vi "DHE_TP.vi"(0 "refnum":i32, 5 "Command":string, 7 "physical unit":string, 9 "swhitches":string[](array[string]), 11 "error in (no error)":errorcluster, 12 "switch arguments":string[](array[string]), 13 "Database RefNum in":T1) -> (4 "refnum out":i32, 6 "response":string, 15 "error out":errorcluster)   [LabVIEW 2016]
uses:
  DBSHAND/private/vis/DatabaseHand_RefNum.ctl
  DHE_TP_action.ctl
panel:
  in  "suscribed?":bool
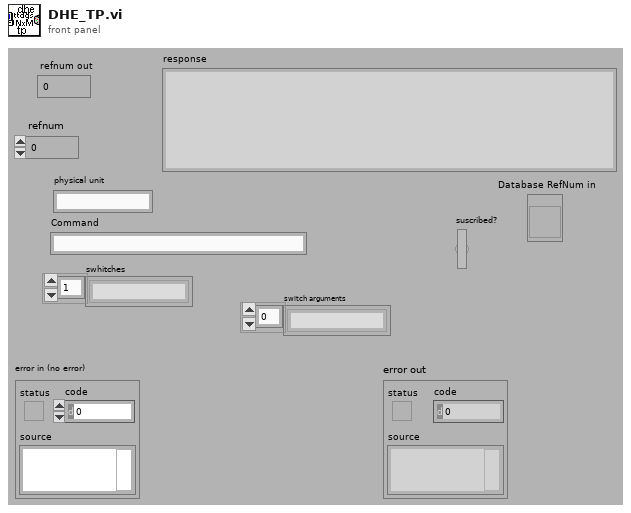
[diagram p1: front panel]
types:
  T1 = typedef "DatabaseHand_RefNum.ctl" = refnum<vi>
  T2 = typedef "DHE_TP_action.ctl" = enum16{"READ FROM FILE", "GET ALL", "FIND BY NAME", "FIND BY TYPE", "SET VALUE", "CLEAN", "CHANGE", "GET EXPUPDATE"}
  T3 = enum16{"convert", "read from file", "get", "clear all", "get all"}
  T4 = enum16{"convert", "read from file", "get", "clear all", "get all", "delete"}
  T5 = typedef "CMN_ContStatus.ctl" = cluster{"Response":string, "power":bool, "shutter":bool, "artifdata":bool, "idlemode":bool, "reset":bool, "gain":u8, "speed":u8, "resetPCI":bool, "autoshutter":bool, "TempSetPoint":i32, "multipleextensions":bool, "displayImage":bool, "coadding":bool, "images being coadded":i32, "Operation Mode":enum16{"normal", "coadd", "fawler"}, "frames to write":cluster{"subs":bool, "reset":bool, "exposed":bool}, "fawler samples":i32, "write auto":bool, "datatype":string, "frames to display":cluster{"subs":bool, "reset":bool, "exposed":bool}, "sur":i32, "autoclear":bool}
  T6 = enum16{"Idle", "Exposing", "Paused", "AbortExp", "Reading", "AbortRead", "FinishedReading", "Resetting", "Reducing", "Initializing"}
  T7 = typedef "DHE_TP.ctl" = cluster{"name":string, "type":string, "R_algor":string[], "board":string, "memory":string, "address":i32, "value":string, "Limits":T8, "unit":string, "params":string, "permissions":string, "W_algor":string[], "description":string, "err_count":i32, "max_err":i32, "read":bool, "lowrej":dbl, "hirej":dbl, "expupd":bool}
  T8 = typedef "DHE_TPLimits.ctl" = cluster{"upper":dbl, "Lower":dbl, "InRange":bool, "nominal":dbl}
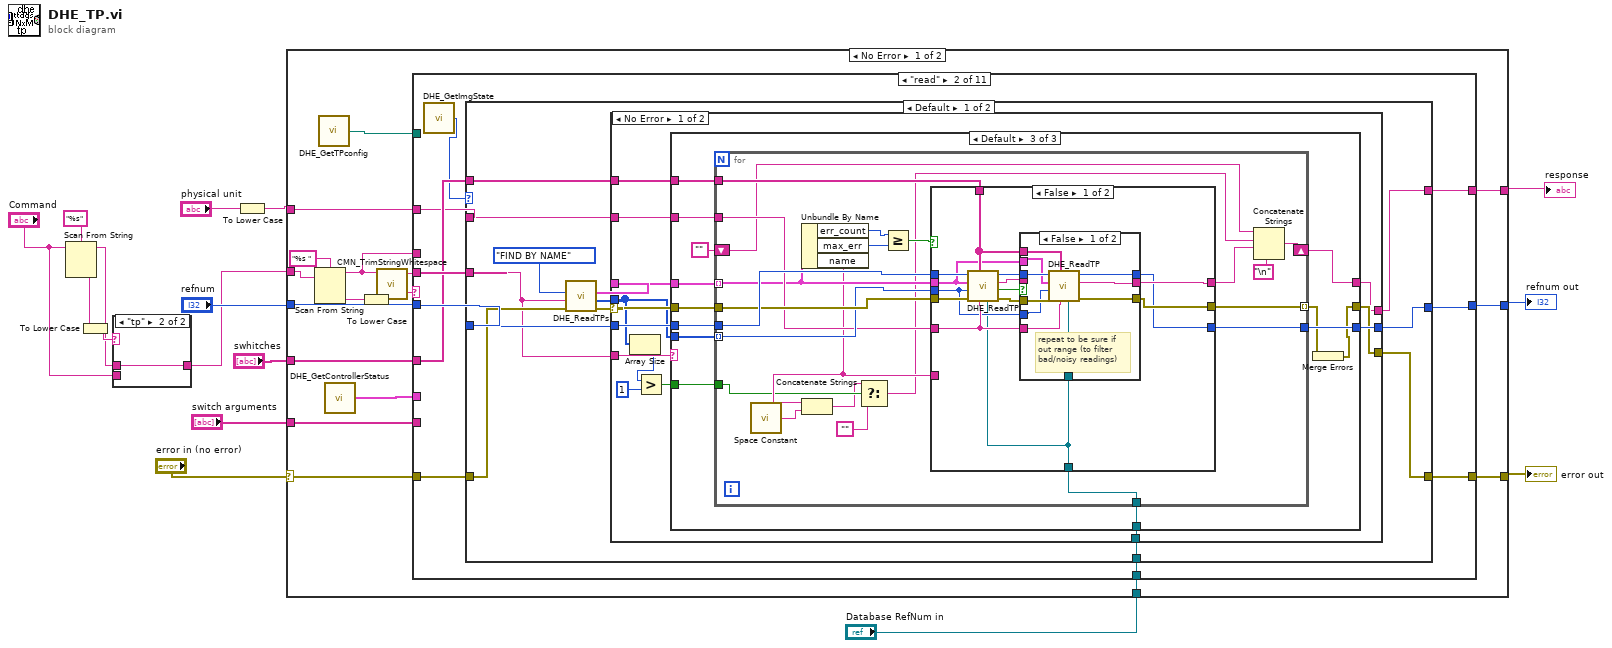
[diagram p0: block diagram]
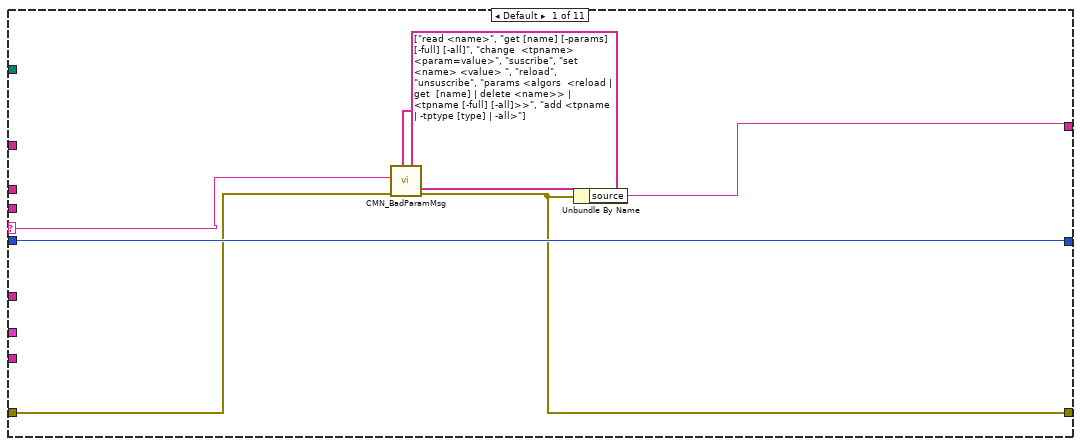
[diagram p3: hidden frame]
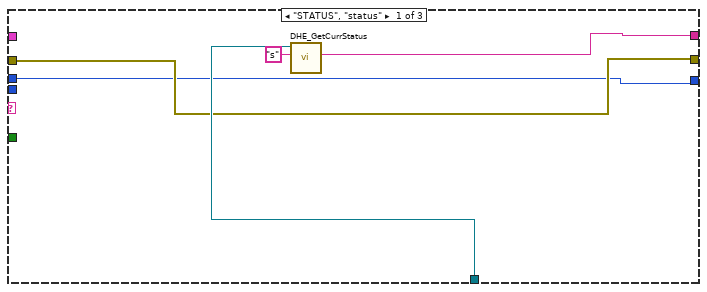
[diagram p4: hidden frame]
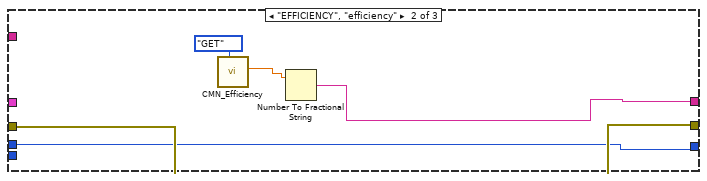
[diagram p5: hidden frame]
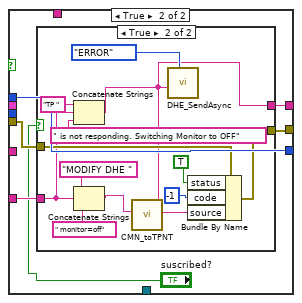
[diagram p7: hidden frame]
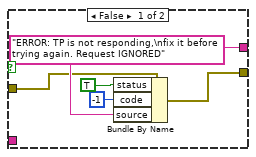
[diagram p8: hidden frame]
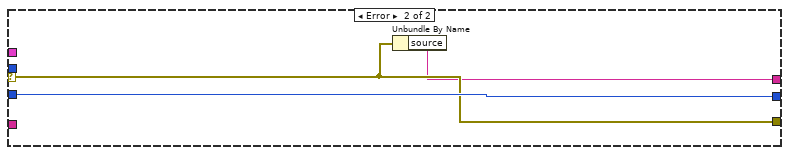
[diagram p9: hidden frame]
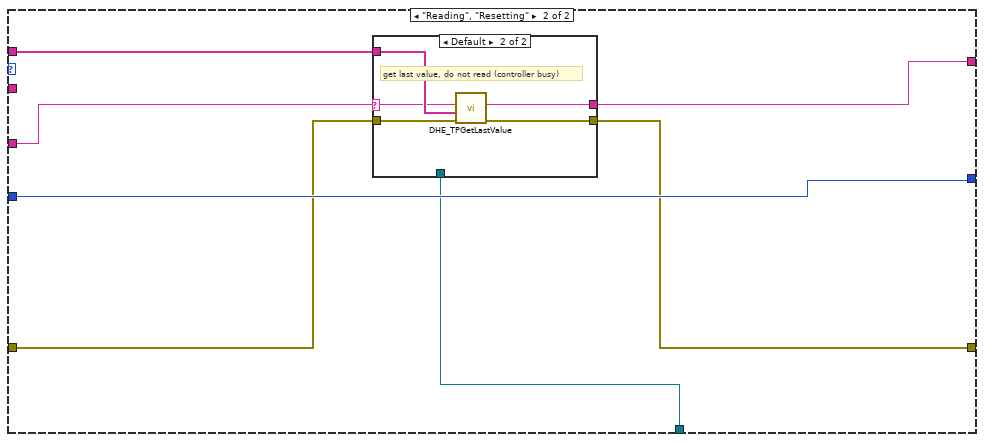
[diagram p10: hidden frame]
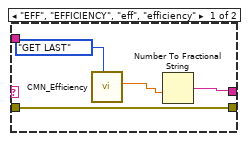
[diagram p11: hidden frame]
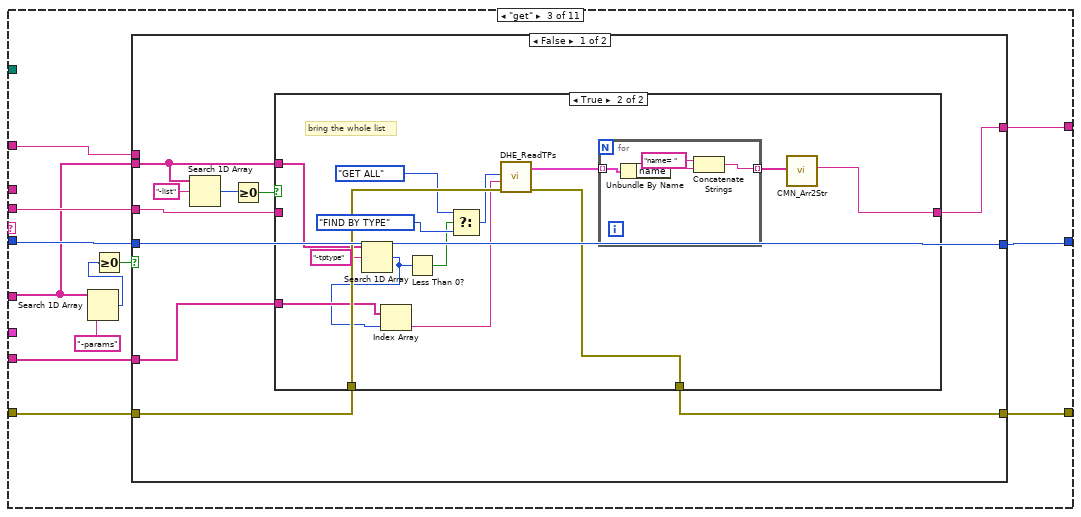
[diagram p12: hidden frame]
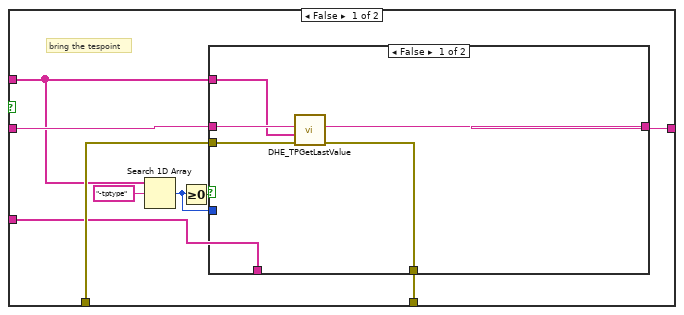
[diagram p13: hidden frame]
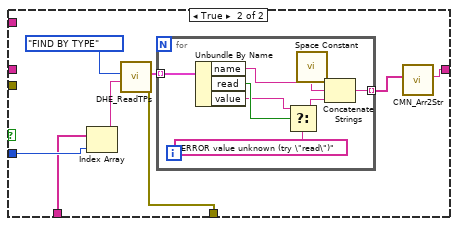
[diagram p14: hidden frame]
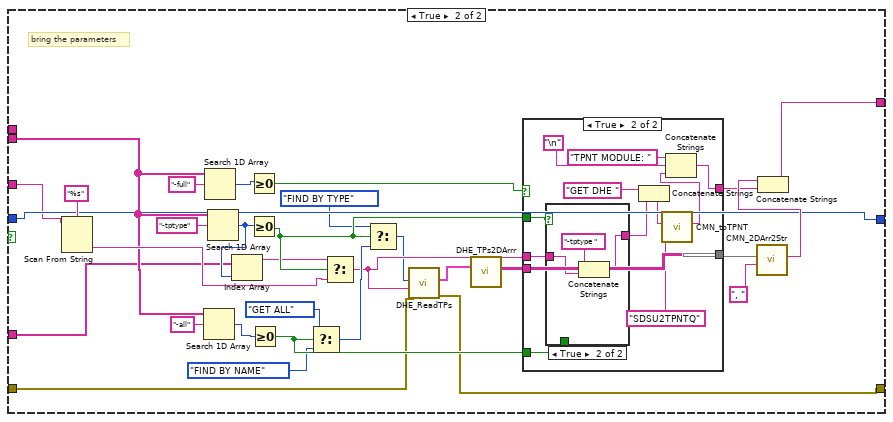
[diagram p15: hidden frame]
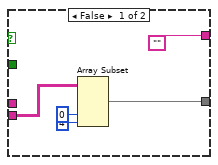
[diagram p16: hidden frame]
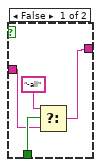
[diagram p17: hidden frame]
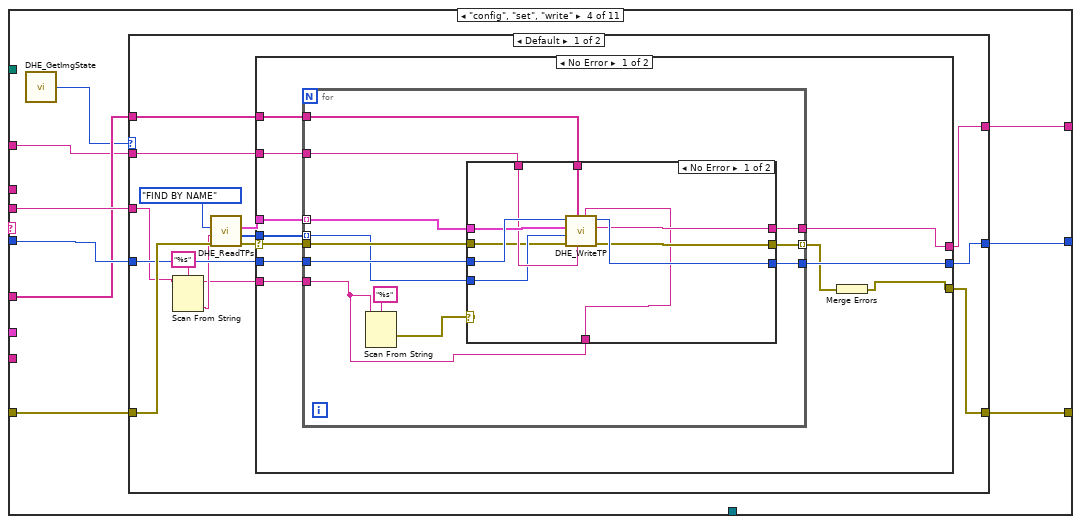
[diagram p18: hidden frame]
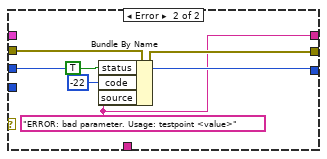
[diagram p19: hidden frame]
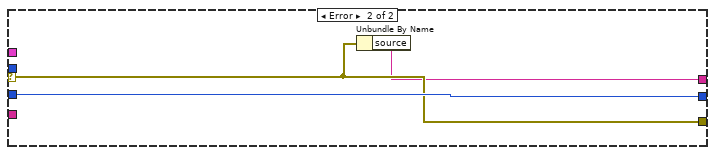
[diagram p20: hidden frame]
diagram:
  n1 = Scan From String(format string="%s", input string="Command") -> (remaining string=w3:string, output 1=w5:string)  [unwired: 2 in, 3 out]
  n2 = To Lower Case(string=w5) -> (all lower case string=w4:string)
  n3 = case shown="\"tp\"" w4 {
    tunnel: w3 -> [_ w18]
    tunnel: [w17 w18] -> w2
    tunnel: "Command" -> [w17 _]
    frame Default {
    }
    frame "tp" {
    }
  }
  n4 = To Lower Case(string="physical unit") -> (all lower case string=w12:string)
  n5 = case shown="No Error" "error in (no error)" {
    selector: "error in (no error)" -> [w22 w635]
    tunnel: [w35 w635] -> w14
    tunnel: "refnum" -> [w34 w637]
    tunnel: [w33 w637] -> w16
    tunnel: w2 -> [w26 _]
    tunnel: w12 -> [w25 _]
    tunnel: [w24 w636] -> w11
    tunnel: "swhitches" -> [w23 _]
    tunnel: "switch arguments" -> [w21 _]
    tunnel: "Database RefNum in" -> [w20 _]
    frame No Error {
      n6 = Scan From String(format string="%s " ("Format String"), input string=w26) -> (remaining string=w28:string, output 1=w29:string)  [unwired: 2 in, 3 out]
      n7 = call "DHE_GetTPconfig.vi"() -> ("DHE_TPcfg"=w19:path)  [unwired: 9 out]
      n8 = call "DHE_GetControllerStatus.vi"() -> ("ControllerStatus"=w27:T5)  [unwired: 11 out]
      n9 = To Lower Case(string=w29) -> (all lower case string=w30:string)
      n10 = call "CMN_TrimStringWhitespace.vi"("string"=w28) -> ("trimmed string"=w31:string)  [unwired: 1 in, 8 out]
      n11 = case shown="\"read\"" w30 {
        selector: w30 -> [w39 _ _ _ _ _ _ _ _ _ _]
        tunnel: w22 -> [w40 w50 w194 w325 _ w461 w472 w481 w505 w609 w634]
        tunnel: [w38 w48 w193 w323 w395 w454 w466 w478 w504 w594 w634] -> w35
        tunnel: w34 -> [w41 w46 w197 w321 w396 w460 w471 w493 w503 w608 w633]
        tunnel: [w41 w49 w204 w324 w396 w460 w471 w493 w503 w608 w633] -> w33
        tunnel: w31 -> [_ w51 w198 w326 w408 w462 _ _ w500 w593 _]
        tunnel: w27 -> [_ _ _ _ _ _ _ _ _ _ _]
        tunnel: w28 -> [_ _ _ _ _ _ _ _ _ _ _]
        tunnel: w25 -> [_ w44 w199 w319 _ _ _ _ _ _ _]
        tunnel: [w37 w47 w203 w322 w391 w459 w464 w492 w501 w607 "module= DHE, prefix= DHE TP, updatecapable= yes, hardware=  DHE hardware controller"] -> w24
        tunnel: w23 -> [_ w45 w196 w320 w399 _ _ _ w502 w598 _]
        tunnel: w21 -> [_ _ w195 _ w398 _ _ _ w506 w610 _]
        tunnel: w19 -> [_ _ _ _ _ _ w473 w479 _ _ _]
        tunnel: w20 -> [_ w43 _ _ _ _ _ _ _ _ _]
        frame Default {
          n12 = call "CMN_BadParamMsg.vi"("valid params"=string[] ["read <name>", "get [name] [-params] [-full] [-all]", "change  <tpname> <param=value>", "suscribe", "set <name> <value> ", "reload", "unsuscribe", "params <algors  <reload | get  [name] | delete <name>> | <tpname [-full] [-all]>>", "add <tpname | -tptype [type] | -all>"], "error in (no error)"=w40, "parameter"=w39) -> ("error out"=w38:errorcluster)  [unwired: 1 in, 7 out]
          n13 = Unbundle By Name(w38) -> ("source"=w37:string)
        }
        frame "read" {
          n14 = call "DHE_GetImgState.vi"() -> ("DHE_ImgState"=w42:T6)  [unwired: 9 out]
          n15 = case shown="Default" w42 {
            tunnel: w51 -> [w53 w178]
            tunnel: w50 -> [w64 w181]
            tunnel: [w63 w183] -> w49
            tunnel: [w62 w180] -> w48
            tunnel: [w61 w179] -> w47
            tunnel: w46 -> [w60 w183]
            tunnel: w45 -> [w59 w182]
            tunnel: w44 -> [w58 _]
            tunnel: w43 -> [w57 w177]
            frame Default {
              n16 = call "DHE_ReadTPs.vi"("error in (no error)"=w64, "argument"=w53, "action"=DHE_TP_action."FIND BY NAME") -> ("error out"=w56:errorcluster, "index"=w54:i32[], "TPs"=w55:T7[])  [unwired: 4 in, 2 out]
              n17 = case shown="No Error" w56 {
                selector: w56 -> [w76 w175]
                tunnel: w55 -> [w74 _]
                tunnel: w60 -> [w78 w176]
                tunnel: [w77 w176] -> w63
                tunnel: [w75 w175] -> w62
                tunnel: [w73 w174] -> w61
                tunnel: w59 -> [w72 _]
                tunnel: w58 -> [w71 _]
                tunnel: w54 -> [w68 _]
                tunnel: w57 -> [w70 _]
                tunnel: w53 -> [w69 _]
                frame No Error {
                  n18 = Array Size(array=w68) -> (size(s)=w67:i32)
                  n19 = Greater?(x=w67, y=1) -> (0:w65:bool)
                  n20 = case shown="Default" w69 {
                    tunnel: w78 -> [w79 w87 w101]
                    tunnel: [w79 w87 w100] -> w77
                    tunnel: w76 -> [w80 w88 w99]
                    tunnel: [w80 w88 w92] -> w75
                    tunnel: w74 -> [_ _ w98]
                    tunnel: w68 -> [_ _ w97]
                    tunnel: [w81 w84 w91] -> w73
                    tunnel: w72 -> [_ _ w96]
                    tunnel: w71 -> [_ _ w95]
                    tunnel: w70 -> [w83 _ w94]
                    tunnel: w65 -> [_ _ w89]
                    frame "STATUS", "status" {
                      n21 = call "DHE_GetCurrStatus.vi"("phys. unit"="s", "Databse Ref"=w83) -> ("progress"=w81:string)  [unwired: 9 out]
                    }
                    frame "EFFICIENCY", "efficiency" {
                      n22 = call "CMN_Efficiency.vi"("Action"=enum16{"ADD", "CLEAR", "GET"}."GET") -> ("efficency"=w85:dbl)  [unwired: 3 in, 7 out]
                      n23 = Number To Fractional String(number=w85) -> (F-format string=w84:string)  [unwired: 3 out]
                    }
                    frame Default {
                      n24 = for {
                        tunnel: w101 -> [w123]
                        tunnel: [w109] -> w100
                        tunnel: w99 -> [w122]
                        tunnel: [w121] -> w93 mode=indexing
                        tunnel: w98 -> [w113] mode=indexing
                        tunnel: w97 -> [w120] mode=indexing
                        tunnel: w96 -> [w119]
                        tunnel: w95 -> [w118]
                        tunnel: w94 -> [w114]
                        shift-right: [w110] -> w91
                        shift-left: "" -> [w108]
                        tunnel: w89 -> [w105]
                        n25 = call <vilib>:"Space Constant.vi"() -> ("String"=w106:string)
                        n26 = Unbundle By Name(w113) -> ("err_count"=w117:i32, "max_err"=w116:i32, "name"=w107:string)
                        n27 = Concatenate Strings(w107, w106) -> (w104:string)
                        n28 = Select(t=w104, s=w105, f="") -> (s? t:f=w102:string)
                        n29 = Greater Or Equal?(x=w117, y=w116) -> (x >= y?=w115:bool)
                        n30 = case shown="False" w115 {
                          tunnel: w123 -> [w137 w156]
                          tunnel: [w129 w156] -> w109
                          tunnel: w122 -> [w136 w154]
                          tunnel: [w133 w153] -> w121
                          tunnel: w120 -> [w125 _]
                          tunnel: [w131 w155] -> w112
                          tunnel: w119 -> [w128 _]
                          tunnel: w118 -> [w127 _]
                          tunnel: w113 -> [w126 _]
                          tunnel: w107 -> [_ w152]
                          tunnel: w114 -> [w124 _]
                          frame False {
                            n31 = call "DHE_ReadTP.vi"("Database RefNum in"=w124, "phys. unit"=w127, "switches"=w128, "error in (no error)"=w136, "index in"=w125, "TP In"=w126, "refnum"=w137) -> ("error out"=w134:errorcluster, "In Range?"=w135:bool, "response"=w132:string, "refnum out"=w130:i32)  [unwired: 1 out]
                            n32 = case shown="False" w135 {
                              tunnel: w134 -> [w147 w150]
                              tunnel: [w140 w150] -> w133
                              tunnel: w132 -> [_ w149]
                              tunnel: [w139 w149] -> w131
                              tunnel: w130 -> [w146 w148]
                              tunnel: [w145 w148] -> w129
                              tunnel: w128 -> [w144 _]
                              tunnel: w127 -> [w143 _]
                              tunnel: w126 -> [w142 _]
                              tunnel: w125 -> [w141 _]
                              tunnel: w124 -> [w138 _]
                              frame False {
                                # "repeat to be sure if\nout range (to filter\nbad/noisy readings)"
                                n33 = call "DHE_ReadTP.vi"("Database RefNum in"=w138, "phys. unit"=w143, "switches"=w144, "error in (no error)"=w147, "index in"=w141, "TP In"=w142, "refnum"=w146) -> ("error out"=w140:errorcluster, "response"=w139:string, "refnum out"=w145:i32)  [unwired: 2 out]
                              }
                              frame True {
                              }
                            }
                          }
                          frame True {
                            n34 = case shown="True" "suscribed?" {
                              tunnel: [w159 w163] -> w155
                              tunnel: w154 -> [w158 w170]
                              tunnel: [w157 w169] -> w153
                              tunnel: w152 -> [_ w162]
                              frame False {
                                w159 = "ERROR: TP is not responding,\nfix it before trying again. Request IGNORED"
                                n35 = Bundle By Name(cluster=w158, "status"=TRUE, "code"=-1, "source"=w159) -> (w157:errorcluster)
                              }
                              frame True {
                                n36 = Concatenate Strings("TP " ("string"), w162, " is not responding. Switching Monitor to OFF" ("Message")) -> (w163:string)
                                n37 = Concatenate Strings("MODIFY DHE " ("string"), w162, " monitor=off" ("string")) -> (w168:string)
                                n38 = call "CMN_toTPNT.vi"("command"=w168) -> ()  [unwired: 3 in, 7 out]
                                n39 = call "DHE_SendAsync.vi"("type"=enum16{"ERROR", "WARNING", "INFO", "CHANGED"}."ERROR", "Message"=w163) -> ()  [unwired: 2 in, 8 out]
                                n40 = Bundle By Name(cluster=w170, "status"=TRUE, "code"=-1, "source"=w163) -> (w169:errorcluster)
                              }
                            }
                          }
                        }
                        n41 = Concatenate Strings(w108, w102, w112, "\n") -> (w110:string)
                      }
                      n42 = Merge Errors(w93) -> (w92:errorcluster)
                    }
                  }
                }
                frame Error {
                  n43 = Unbundle By Name(w175) -> ("source"=w174:string)
                }
              }
            }
            frame "Reading", "Resetting" {
              n44 = case shown="Default" w178 {
                selector: w178 -> [_ w188]
                tunnel: w182 -> [_ w192]
                tunnel: w181 -> [w187 w191]
                tunnel: [w187 w190] -> w180
                tunnel: [w185 w189] -> w179
                tunnel: w177 -> [_ _]
                frame "EFF", "EFFICIENCY", "eff", "efficiency" {
                  n45 = call "CMN_Efficiency.vi"("Action"=enum16{"ADD", "CLEAR", "GET", "GET LAST"}."GET LAST") -> ("efficency"=w186:dbl)  [unwired: 3 in, 7 out]
                  n46 = Number To Fractional String(number=w186) -> (F-format string=w185:string)  [unwired: 3 out]
                }
                frame Default {
                  # "get last value, do not read (controller busy)"
                  n47 = call "DHE_TPGetLastValue.vi"("error in (no error)"=w191, "swhitches"=w192, "name"=w188) -> ("error IO"=w190:errorcluster, "value"=w189:string)  [unwired: 7 out]
                }
              }
            }
          }
        }
        frame "get" {
          n48 = Search 1D Array(1D array=w196, element="-params") -> (index of element=w200:i32)  [unwired: 1 out]
          n49 = Greater Or Equal To 0?(x=w200) -> (x >= 0?=w201:bool)
          n50 = case shown="False" w201 {
            tunnel: w198 -> [w213 w271]
            tunnel: w194 -> [w212 w274]
            tunnel: [w214 w272] -> w204
            tunnel: [w211 w273] -> w193
            tunnel: [w210 w269] -> w203
            tunnel: w197 -> [w214 w272]
            tunnel: w199 -> [_ _]
            tunnel: w196 -> [w209 w268]
            tunnel: w195 -> [w205 w267]
            frame False {
              n51 = Search 1D Array(1D array=w209, element="-list") -> (index of element=w207:i32)  [unwired: 1 out]
              n52 = Greater Or Equal To 0?(x=w207) -> (x >= 0?=w206:bool)
              n53 = case shown="True" w206 {
                tunnel: w213 -> [w223 _]
                tunnel: w212 -> [w222 w257]
                tunnel: [w221 w256] -> w211
                tunnel: w209 -> [w218 w253]
                tunnel: [w220 w254] -> w210
                tunnel: w205 -> [w215 w251]
                frame False {
                  # "bring the tespoint"
                  n54 = Search 1D Array(1D array=w218, element="-tptype") -> (index of element=w216:i32)  [unwired: 1 out]
                  n55 = Greater Or Equal To 0?(x=w216) -> (x >= 0?=w217:bool)
                  n56 = case shown="False" w217 {
                    tunnel: w223 -> [w228 _]
                    tunnel: w222 -> [w227 _]
                    tunnel: [w226 w232] -> w221
                    tunnel: [w225 w229] -> w220
                    tunnel: w218 -> [w224 _]
                    tunnel: w216 -> [_ w236]
                    tunnel: w215 -> [_ w235]
                    frame False {
                      n57 = call "DHE_TPGetLastValue.vi"("error in (no error)"=w227, "swhitches"=w224, "name"=w228) -> ("error IO"=w226:errorcluster, "value"=w225:string)  [unwired: 7 out]
                    }
                    frame True {
                      n58 = Index Array(array=w235, index=w236) -> (element=w233:string)
                      n59 = call "DHE_ReadTPs.vi"("argument"=w233, "action"=DHE_TP_action."FIND BY TYPE") -> ("error out"=w232:errorcluster, "TPs"=w231:T7[])  [unwired: 5 in, 3 out]
                      n60 = for {
                        tunnel: w231 -> [w244] mode=indexing
                        tunnel: [w241] -> w230 mode=indexing
                        n61 = Unbundle By Name(w244) -> ("name"=w243:string, "read"=w240:bool, "value"=w239:string)
                        n62 = Select(t=w239, s=w240, f="ERROR value unknown (try \"read\")") -> (s? t:f=w238:string)
                        n63 = call <vilib>:"Space Constant.vi"() -> ("String"=w242:string)
                        n64 = Concatenate Strings(w243, w242, w238) -> (w241:string)
                      }
                      n65 = call "CMN_Arr2Str.vi"("Array in"=w230) -> ("string out"=w229:string)  [unwired: 10 out]
                    }
                  }
                }
                frame True {
                  # "bring the whole list"
                  n66 = Search 1D Array(1D array=w253, element="-tptype") -> (index of element=w250:i32)  [unwired: 1 out]
                  n67 = Index Array(array=w251, index=w250) -> (element=w249:string)
                  n68 = Less Than 0?(x=w250) -> (x < 0?=w245:bool)
                  n69 = Select(t=DHE_TP_action."GET ALL" ("action"), s=w245, f=DHE_TP_action."FIND BY TYPE" ("action")) -> (s? t:f=w246:T2)
                  n70 = call "DHE_ReadTPs.vi"("error in (no error)"=w257, "argument"=w249, "action"=w246) -> ("error out"=w256:errorcluster, "TPs"=w258:T7[])  [unwired: 4 in, 3 out]
                  n71 = for {
                    tunnel: w258 -> [w262] mode=indexing
                    tunnel: [w259] -> w255 mode=indexing
                    n72 = Unbundle By Name(w262) -> ("name"=w261:string)
                    n73 = Concatenate Strings("name= " ("string"), w261) -> (w259:string)
                  }
                  n74 = call "CMN_Arr2Str.vi"("Array in"=w255) -> ("string out"=w254:string)  [unwired: 10 out]
                }
              }
            }
            frame True {
              # "bring the parameters"
              n75 = Scan From String(format string="%s", input string=w271) -> (output 1=w292:string)  [unwired: 2 in, 4 out]
              n76 = Search 1D Array(1D array=w268, element="-all") -> (index of element=w283:i32)  [unwired: 1 out]
              n77 = Search 1D Array(1D array=w268, element="-full") -> (index of element=w290:i32)  [unwired: 1 out]
              n78 = Search 1D Array(1D array=w268, element="-tptype") -> (index of element=w280:i32)  [unwired: 1 out]
              n79 = Index Array(array=w267, index=w280) -> (element=w270:string)
              n80 = Greater Or Equal To 0?(x=w290) -> (x >= 0?=w289:bool)
              n81 = Greater Or Equal To 0?(x=w280) -> (x >= 0?=w279:bool)
              n82 = Greater Or Equal To 0?(x=w283) -> (x >= 0?=w277:bool)
              n83 = Select(t=DHE_TP_action."GET ALL" ("action"), s=w277, f=DHE_TP_action."FIND BY NAME" ("action")) -> (s? t:f=w281:T2)
              n84 = Select(t=w270, s=w279, f=w292) -> (s? t:f=w278:string)
              n85 = Select(t=DHE_TP_action."FIND BY TYPE" ("action"), s=w279, f=w281) -> (s? t:f=w263:T2)
              n86 = call "DHE_ReadTPs.vi"("error in (no error)"=w274, "argument"=w278, "action"=w263) -> ("error out"=w273:errorcluster, "TPs"=w288:T7[])  [unwired: 4 in, 3 out]
              n87 = call "DHE_TPs2DArrr.vi"("TPs"=w288) -> ("TPs out"=w287:string[][])  [unwired: 10 out]
              n88 = case shown="True" w289 {
                tunnel: w287 -> [w298 w310]
                tunnel: [w295 w310] -> w286
                tunnel: w279 -> [_ w309]
                tunnel: w278 -> [_ w306]
                tunnel: w277 -> [_ w304]
                tunnel: ["" w301] -> w275
                frame False {
                  n89 = Array Subset(array=w298, index (col)=0 ("index"), length (col)=4 ("length")) -> (w295:string[][])  [unwired: 2 in]
                }
                frame True {
                  n90 = case shown="True" w309 {
                    tunnel: w306 -> [w311 w316]
                    tunnel: [w312 w315] -> w305
                    tunnel: w304 -> [w314 _]
                    frame False {
                      n91 = Select(t="-all", s=w314, f=w311) -> (s? t:f=w312:string)
                    }
                    frame True {
                      n92 = Concatenate Strings("-tptype ", w316) -> (w315:string)
                    }
                  }
                  n93 = Concatenate Strings("GET DHE " ("command"), w305) -> (w307:string)
                  n94 = call "CMN_toTPNT.vi"("respond to"="SDSU2TPNTQ", "command"=w307) -> ("reply"=w302:string)  [unwired: 2 in, 6 out]
                  n95 = Concatenate Strings("TPNT MODULE: " ("string"), "\n", w302) -> (w301:string)
                }
              }
              n96 = call "CMN_2DArr2Str.vi"("separator"=", ", "array in"=w286) -> ("string out"=w276:string)  [unwired: 9 out]
              n97 = Concatenate Strings(w276, w275) -> (w269:string)
            }
          }
        }
        frame "config", "set", "write" {
          n98 = call "DHE_GetImgState.vi"() -> ("DHE_ImgState"=w318:T6)  [unwired: 9 out]
          n99 = case shown="Default" w318 {
            tunnel: w326 -> [w331 _]
            tunnel: w325 -> [w341 w388]
            tunnel: [w338 w389] -> w324
            tunnel: [w337 w385] -> w323
            tunnel: [w336 w384] -> w322
            tunnel: w321 -> [w335 w389]
            tunnel: w320 -> [w334 _]
            tunnel: w319 -> [w333 _]
            frame Default {
              n100 = Scan From String(format string="%s", input string=w331) -> (remaining string=w328:string, output 1=w329:string)  [unwired: 2 in, 3 out]
              n101 = call "DHE_ReadTPs.vi"("error in (no error)"=w341, "argument"=w329, "action"=DHE_TP_action."FIND BY NAME") -> ("error out"=w340:errorcluster, "index"=w332:i32[], "TPs"=w339:T7[])  [unwired: 4 in, 2 out]
              n102 = case shown="No Error" w340 {
                selector: w340 -> [w350 w382]
                tunnel: w339 -> [w348 _]
                tunnel: w335 -> [w352 w383]
                tunnel: [w351 w383] -> w338
                tunnel: [w342 w382] -> w337
                tunnel: [w349 w381] -> w336
                tunnel: w334 -> [w347 _]
                tunnel: w333 -> [w346 _]
                tunnel: w332 -> [w345 _]
                tunnel: w328 -> [w344 _]
                frame No Error {
                  n103 = for {
                    tunnel: w352 -> [w364]
                    tunnel: [w363] -> w351
                    tunnel: w350 -> [w362]
                    tunnel: [w361] -> w349
                    tunnel: w348 -> [w354] mode=indexing
                    tunnel: w347 -> [w360]
                    tunnel: w346 -> [w359]
                    tunnel: w345 -> [w358] mode=indexing
                    tunnel: w344 -> [w355]
                    tunnel: [w353] -> w343 mode=indexing
                    n104 = Scan From String(format string="%s", input string=w355) -> (error out=w356:errorcluster)  [unwired: 2 in, 4 out]
                    n105 = case shown="No Error" w356 {
                      tunnel: w364 -> [w374 w376]
                      tunnel: [w373 w376] -> w363
                      tunnel: w362 -> [w365 w380]
                      tunnel: [w372 w377] -> w353
                      tunnel: [w371 w375] -> w361
                      tunnel: w354 -> [w370 _]
                      tunnel: w360 -> [w369 _]
                      tunnel: w359 -> [w368 _]
                      tunnel: w358 -> [w367 _]
                      tunnel: w355 -> [w366 _]
                      frame No Error {
                        n106 = call "DHE_WriteTP.vi"("value"=w366, "phys. unit"=w368, "switches"=w369, "error in (no error)"=w365, "index in"=w367, "TP In"=w370, "refnum"=w374) -> ("error out"=w372:errorcluster, "response"=w371:string, "refnum out"=w373:i32)  [unwired: 2 out]
                      }
                      frame Error {
                        w375 = "ERROR: bad parameter. Usage: testpoint <value>" ("source")
                        n107 = Bundle By Name(cluster=w380, "status"=TRUE, "code"=-22, "source"=w375) -> (w377:errorcluster)
                      }
                    }
                  }
                  n108 = Merge Errors(w343) -> (w342:errorcluster)
                }
                frame Error {
                  n109 = Unbundle By Name(w382) -> ("source"=w381:string)
                }
              }
            }
            frame "Exposing", "Reading", "Resetting" {
              w384 = "WARNING: controller busy -testpoint NOT READ" ("source")
              n110 = Bundle By Name(cluster=w388, "status"=FALSE, "code"=-1, "source"=w384) -> (w385:errorcluster)
            }
          }
        }
        frame "add" {
          n111 = Scan From String(format string="%s", input string=w408) -> (output 1=w397:string)  [unwired: 2 in, 4 out]
          n112 = Search 1D Array(1D array=w399, element="-all") -> (index of element=w405:i32)  [unwired: 1 out]
          n113 = To Lower Case(string=w397) -> (all lower case string=w404:string)
          n114 = Greater Or Equal To 0?(x=w405) -> (x >= 0?=w401:bool)
          n115 = Equal?(x=w404, y="all") -> (x = y?=w402:bool)
          n116 = Or(x=w402, y=w401) -> (x .or. y?=w400:bool)
          n117 = case shown="True" w400 {
            tunnel: [w440 DHE_TP_action."GET ALL" ("action")] -> w390
            tunnel: w399 -> [w441 _]
            tunnel: w398 -> [w439 _]
            tunnel: [w437 ""] -> w392
            tunnel: w397 -> [w436 _]
            frame False {
              n118 = Search 1D Array(1D array=w441, element="-tptype") -> (index of element=w438:i32)  [unwired: 1 out]
              n119 = Greater Or Equal To 0?(x=w438) -> (x >= 0?=w435:bool)
              n120 = case shown="False" w435 {
                tunnel: [DHE_TP_action."FIND BY NAME" ("action") DHE_TP_action."FIND BY TYPE" ("action")] -> w440
                tunnel: w439 -> [_ w448]
                tunnel: w438 -> [_ w447]
                tunnel: [w444 w446] -> w437
                tunnel: w436 -> [w444 _]
                frame False {
                }
                frame True {
                  n121 = Index Array(array=w448, index=w447) -> (element=w446:string)
                }
              }
            }
            frame True {
            }
          }
          n122 = call "DHE_ReadTPs.vi"("argument"=w392, "action"=w390) -> ("error out"=w393:errorcluster, "TPs"=w394:T7[])  [unwired: 5 in, 3 out]
          n123 = case shown="No Error" w393 {
            selector: w393 -> [_ w434]
            tunnel: [w411 w434] -> w395
            tunnel: [w410 w433] -> w391
            tunnel: w394 -> [w409 _]
            frame No Error {
              n124 = for {
                tunnel: w409 -> [w432] mode=indexing
                tunnel: [w428] -> w412 mode=indexing
                tunnel: [w427] -> w410
                n125 = Unbundle By Name(w432) -> ("permissions"=w415:string, "name"=w425:string, "type"=w424:string, "Limits.Lower"=w423:dbl, "Limits.nominal"=w422:dbl, "Limits.upper"=w421:dbl, "params"=w418:string)
                n126 = Empty String/Path?(string/path=w418) -> (empty?=w420:bool)
                n127 = Concatenate Strings("," ("string"), w418) -> (w416:string)
                n128 = Select(t="", s=w420, f=w416) -> (s? t:f=w414:string)
                n129 = Format Into String(format string="name=%s, type=%s, range=%g %g %g, permissions=%s %s", initial string="ADD DHE " ("format string"), w425, w424, w423, w422, w421, w415, w414) -> (resulting string=w430:string)  [unwired: 1 in, 1 out]
                n130 = call "CMN_toTPNT.vi"("timeout"=30, "respond to"="DHE_TPNTQ", "command"=w430) -> ("error out"=w428:errorcluster, "reply"=w427:string)  [unwired: 1 in, 5 out]
              }
              n131 = call "CMN_CombineErrors.vi"("Errors"=w412) -> ("error out"=w411:errorcluster)  [unwired: 10 out]
            }
            frame Error {
              n132 = Unbundle By Name(w434) -> ("source"=w433:string)
            }
          }
        }
        frame "delete", "unsuscribe" {
          n133 = Scan From String(format string="%s", input string=w462) -> (output 1=w456:string)  [unwired: 2 in, 4 out]
          n134 = Concatenate Strings("DELETE DHE " ("format string"), w456) -> (w455:string)
          n135 = call "CMN_toTPNT.vi"("error in (no error)"=w461, "command"=w455) -> ("error out"=w454:errorcluster, "reply"=w459:string)  [unwired: 2 in, 5 out]
          n136 = property on="suscribed?" class="Bool (strict)"() -> ("Value"=w453:bool)  [unwired: 2 in, 2 out]
          n137 = Select(t=w453, s=w454, f=FALSE) -> (s? t:f=w452:bool)
          n138 = property on="suscribed?" class="Bool (strict)"("Value"=w452) -> ()  [unwired: 2 in, 2 out]
        }
        frame "reload" {
          n139 = call "DHE_ReadTPs.vi"("error in (no error)"=w472, "action"=DHE_TP_action."READ FROM FILE", "file path"=w473) -> ("error out"=w466:errorcluster, "TPs"=w470:T7[])  [unwired: 4 in, 3 out]
          n140 = Array Size(array=w470) -> (size(s)=w469:i32)
          n141 = Format Into String(format string="DONE: reloaded %d points", w469) -> (resulting string=w465:string)  [unwired: 2 in, 1 out]
          n142 = Unbundle By Name(w466) -> ("source"=w467:string)
          n143 = Select(t=w467, s=w466, f=w465) -> (s? t:f=w464:string)
        }
        frame "subscribe", "suscribe" {
          n144 = call "DHE_ReadTPs.vi"("action"=DHE_TP_action."READ FROM FILE", "file path"=w479) -> ("devparams"=w486:string)  [unwired: 5 in, 4 out]
          n145 = Empty String/Path?(string/path=w486) -> (empty?=w489:bool)
          n146 = call "DHE_StartTPNT.vi"("error in (no error)"=w481) -> ("error out"=w482:errorcluster)  [unwired: 10 out]
          n147 = Concatenate Strings("," ("string"), w486) -> (w484:string)
          n148 = stacked-sequence {
            tunnel: w482 -> [_]
            tunnel: [w496] -> w480
            tunnel: w481 -> [w496]
            frame #0 {
              n149 = call "CMN_toTPNT.vi"("timeout"=4000, "command"="STATE") -> ()  [unwired: 2 in, 7 out]
            }
          }
          n150 = Select(t="", s=w489, f=w484) -> (s? t:f=w487:string)
          n151 = Concatenate Strings("SUSCRIBE DHE FORCE interface=PAN DHE  TP" ("format string"), w487) -> (w483:string)
          n152 = call "CMN_toTPNT.vi"("timeout"=3000, "error in (no error)"=w480, "respond to"="DHE_TPNTQ", "command"=w483) -> ("error out"=w478:errorcluster, "reply"=w492:string)  [unwired: 5 out]
          n153 = Unbundle By Name(w478) -> ("status"=w477:bool)
          n154 = Not(x=w477) -> (.not. x?=w476:bool)
          n155 = property on="suscribed?" class="Bool (strict)"("Value"=w476) -> ()  [unwired: 2 in, 2 out]
        }
        frame "definition", "parameters", "params", "testpoints" {
          n156 = Scan From String(format string="%s", input string=w500) -> (remaining string=w497:string, output 1=w498:string)  [unwired: 2 in, 3 out]
          n157 = case shown="Default" w498 {
            selector: w498 -> [_ w554]
            tunnel: w506 -> [_ w552]
            tunnel: w505 -> [w517 w568]
            tunnel: [w516 w567] -> w504
            tunnel: w502 -> [_ w556]
            tunnel: [w518 w547] -> w501
            tunnel: w497 -> [w515 _]
            frame "algors" {
              n158 = Scan From String(format string="%s", input string=w515) -> (remaining string=w510:string, output 1=w513:string)  [unwired: 2 in, 3 out]
              n159 = To Lower Case(string=w513) -> (all lower case string=w512:string)
              n160 = call "CMN_TrimStringWhitespace.vi"("string"=w510) -> ("trimmed string"=w509:string)  [unwired: 1 in, 8 out]
              n161 = case shown="\"get\", Default" w512 {
                tunnel: [w522 T4."delete" ("action") T3."read from file" ("action")] -> w507
                tunnel: w509 -> [w520 w531 w539]
                tunnel: [w521 path "" w535] -> w511
                tunnel: [w519 w530 string[] []] -> w508
                frame "get", Default {
                  n162 = case shown="\"\", \" \", \"-all\", \"all\"" w520 {
                    selector: w520 -> [w524 _]
                    tunnel: [T3."get" ("action") T3."get all" ("action")] -> w522
                    tunnel: [path "" path ""] -> w521
                    tunnel: [w525 string[] []] -> w519
                    frame Default {
                      n163 = Build Array(w524) -> (w525:string[])
                    }
                    frame "", " ", "-all", "all" {
                    }
                  }
                }
                frame "delete" {
                  n164 = Build Array(w531) -> (w530:string[])
                }
                frame "reload" {
                  # "read the default file unless\na diferent one is specified"
                  n165 = String To Path(string=w539) -> (path=w536:path)
                  n166 = Empty String/Path?(string/path=w536) -> (empty?=w537:bool)
                  n167 = call "DHE_GetAlgorsFile.vi"() -> ("DHE_AlgorsFile"=w534:path)  [unwired: 9 out]
                  n168 = Select(t=w534, s=w537, f=w536) -> (s? t:f=w535:path)
                }
              }
              n169 = call "CMN_Algors.vi"("file"=w511, "algors"=w508, "error in (no error)"=w517, "action"=w507) -> ("string value"=w518:string, "error out"=w516:errorcluster)  [unwired: 1 in, 4 out]
            }
            frame Default {
              n170 = Search 1D Array(1D array=w556, element="-all") -> (index of element=w558:i32)  [unwired: 1 out]
              n171 = Search 1D Array(1D array=w556, element="-full") -> (index of element=w565:i32)  [unwired: 1 out]
              n172 = Search 1D Array(1D array=w556, element="-tptype") -> (index of element=w553:i32)  [unwired: 1 out]
              n173 = Index Array(array=w552, index=w553) -> (element=w551:string)
              n174 = Greater Or Equal To 0?(x=w565) -> (x >= 0?=w564:bool)
              n175 = Greater Or Equal To 0?(x=w553) -> (x >= 0?=w550:bool)
              n176 = Greater Or Equal To 0?(x=w558) -> (x >= 0?=w548:bool)
              n177 = Select(t=DHE_TP_action."GET ALL" ("action"), s=w548, f=DHE_TP_action."FIND BY NAME" ("action")) -> (s? t:f=w555:T2)
              n178 = Select(t=w551, s=w550, f=w554) -> (s? t:f=w549:string)
              n179 = Select(t=DHE_TP_action."FIND BY TYPE" ("action"), s=w550, f=w555) -> (s? t:f=w542:T2)
              n180 = call "DHE_ReadTPs.vi"("error in (no error)"=w568, "argument"=w549, "action"=w542) -> ("error out"=w567:errorcluster, "TPs"=w563:T7[])  [unwired: 4 in, 3 out]
              n181 = call "DHE_TPs2DArrr.vi"("TPs"=w563) -> ("TPs out"=w562:string[][])  [unwired: 10 out]
              n182 = case shown="True" w564 {
                tunnel: w562 -> [w573 w585]
                tunnel: [w570 w585] -> w561
                tunnel: w550 -> [_ w584]
                tunnel: w549 -> [_ w581]
                tunnel: w548 -> [_ w579]
                tunnel: ["" w576] -> w545
                frame False {
                  n183 = Array Subset(array=w573, index (col)=0 ("index"), length (col)=4 ("length")) -> (w570:string[][])  [unwired: 2 in]
                }
                frame True {
                  w574 = "\n"
                  n184 = case shown="False" w584 {
                    tunnel: w581 -> [w586 w591]
                    tunnel: [w587 w590] -> w580
                    tunnel: w579 -> [w589 _]
                    frame False {
                      n185 = Select(t="-all", s=w589, f=w586) -> (s? t:f=w587:string)
                    }
                    frame True {
                      n186 = Concatenate Strings("-tptype ", w591) -> (w590:string)
                    }
                  }
                  n187 = Concatenate Strings("GET DHE " ("command"), w580) -> (w582:string)
                  n188 = call "CMN_toTPNT.vi"("respond to"="SDSU2TPNTQ", "command"=w582) -> ("reply"=w577:string)  [unwired: 2 in, 6 out]
                  n189 = Concatenate Strings(w574, "TPNT MODULE: " ("string"), w574, w577) -> (w576:string)
                }
              }
              n190 = call "CMN_2DArr2Str.vi"("separator"=", ", "array in"=w561) -> ("string out"=w546:string)  [unwired: 9 out]
              n191 = Concatenate Strings(w546, w545) -> (w547:string)
            }
          }
        }
        frame "change", "modify" {
          w604 = "-tptype" ("element")
          n192 = Search 1D Array(1D array=w598, element="-all") -> (index of element=w596:i32)  [unwired: 1 out]
          n193 = Search 1D Array(1D array=w598, element=w604) -> (index of element=w602:i32)  [unwired: 1 out]
          n194 = Greater Or Equal To 0?(x=w602) -> (x >= 0?=w603:bool)
          n195 = Greater Or Equal To 0?(x=w596) -> (x >= 0?=w595:bool)
          n196 = case shown="False" w603 {
            tunnel: w602 -> [_ w631]
            tunnel: w610 -> [_ w630]
            tunnel: w604 -> [_ w628]
            tunnel: [w622 w626] -> w600
            tunnel: w595 -> [w625 _]
            frame False {
              n197 = Select(t="-all", s=w625, f="") -> (s? t:f=w622:string)
            }
            frame True {
              n198 = Index Array(array=w630, index=w631) -> (element=w627:string)
              n199 = Concatenate Strings(w628, " " ("string"), w627) -> (w626:string)
            }
          }
          n200 = Concatenate Strings("MODIFY DHE " ("string"), w600, " " ("string"), w593) -> (w605:string)
          n201 = call "CMN_toTPNT.vi"("error in (no error)"=w609, "respond to"="DHE_TPNTQ", "command"=w605) -> ("error out"=w594:errorcluster, "reply"=w607:string)  [unwired: 1 in, 5 out]
          n202 = case shown="No Error" w594 {
            tunnel: w593 -> [w616 _]
            frame No Error {
              n203 = Scan From String(format string="%s", input string=w616) -> (remaining string=w620:string, output 1=w619:string)  [unwired: 2 in, 3 out]
              n204 = call "DHE_ReadTPs.vi"("argument"=w619, "action"=DHE_TP_action."FIND BY NAME") -> ("error out"=w617:errorcluster, "index"=w613:i32[])  [unwired: 5 in, 3 out]
              n205 = call "CMN_TrimStringWhitespace.vi"("string"=w620) -> ("trimmed string"=w621:string)  [unwired: 1 in, 8 out]
              n206 = Index Array(array=w613, index=0) -> (element=w611:i32)
              n207 = call "DHE_ReadTPs.vi"("index in"=w611, "error in (no error)"=w617, "argument"=w621, "action"=DHE_TP_action."CHANGE") -> ()  [unwired: 3 in, 5 out]
            }
            frame Error {
            }
          }
        }
        frame "modinfo" {
        }
      }
    }
    frame Error {
      n208 = Unbundle By Name(w635) -> ("source"=w636:string)  [unwired: 1 out]
    }
  }
  "refnum out" <- w16
  "error out" <- w14
  "response" <- w11
